vi "handle menu selection.vi"(6 "menu ref":refnum<k9>, 9 "ItemTag":string, 10 "ItemPath":string, 11 "Queue in":refnum<queue>) -> (0 "close?":bool=TRUE)   [LabVIEW 2018]
uses:
  queue data type.ctl
  state.ctl
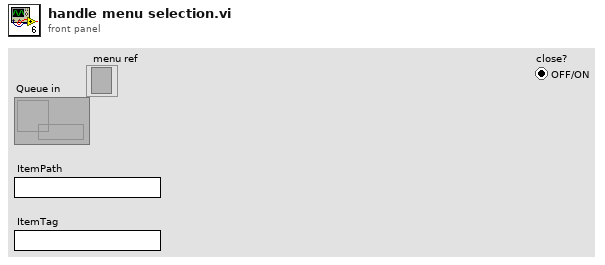
[diagram p1: front panel]
types:
  T1 = typedef "queue data type.ctl" = cluster{"state":T2, "data":variant}
  T2 = typedef "state.ctl" = enum16{"readData", "init", "channel", "mode", "quit"}
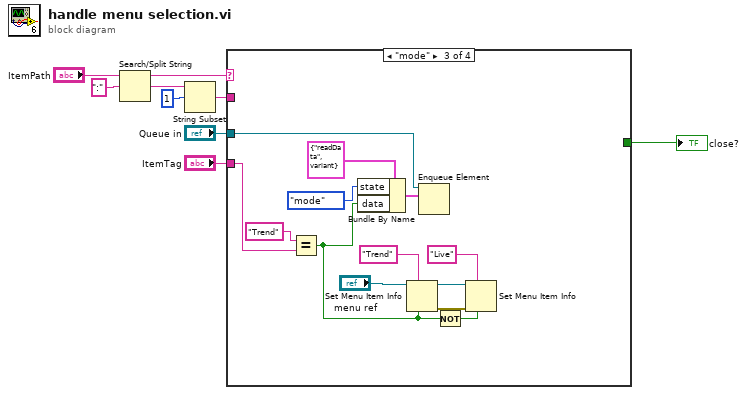
[diagram p0: block diagram]
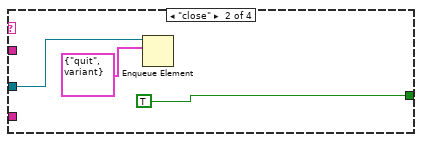
[diagram p3: hidden frame]
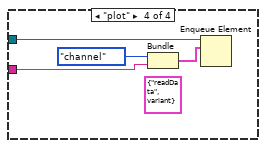
[diagram p4: hidden frame]
diagram:
  n1 = Search/Split String(string="ItemPath", search string/char (-)=":") -> (substring before match=w6:string, match + rest of string=w5:string)  [unwired: 1 in, 1 out]
  n2 = String Subset(string=w5, offset (0)=1) -> (substring=w3:string)  [unwired: 1 in]
  n3 = case shown="\"mode\"" w6 {
    tunnel: w3 -> [_ _ _ _]
    tunnel: "Queue in" -> [_ w11 w25 w27]
    tunnel: "ItemTag" -> [_ _ w24 w26]
    tunnel: [_ TRUE _ _] -> w1
    frame "", Default {
    }
    frame "close" {
      n4 = Enqueue Element(queue=w11, element=T1 {"state"=enum."quit", "data"=variant}) -> ()  [unwired: 2 in, 3 out]
    }
    frame "mode" {
      n5 = Equal?(x="Trend", y=w24) -> (x = y?=w14:bool)
      n6 = Bundle By Name(cluster=T1 {"state"=enum."readData", "data"=variant} ("element"), "state"=state."mode", "data"=w14) -> (w21:T1)
      n7 = Set Menu Item Info(6:w14, 7:"Trend" ("item tag"), 11:"menu ref") -> (0:w17:errorcluster, 3:w16:refnum<k9>)  [unwired: 4 in]
      n8 = Enqueue Element(queue=w25, element=w21) -> ()  [unwired: 2 in, 3 out]
      n9 = Not(x=w14) -> (.not. x?=w13:bool)
      n10 = Set Menu Item Info(6:w13, 7:"Live" ("item tag"), 8:w17, 11:w16) -> ()  [unwired: 3 in, 2 out]
    }
    frame "plot" {
      (unwired) T1 {"state"=enum."readData", "data"=variant} ("cluster")
      n11 = Bundle(state."channel", "ItemTag"=w26) -> (w28:cluster{T2, "ItemTag":string})  [unwired: 1 in]
      n12 = Enqueue Element(queue=w27, element=w28) -> ()  [unwired: 2 in, 3 out]
    }
  }
  "close?" <- w1
